vi "Read Test running.vi"(8 "error in (no error)":errorcluster, 11 "Fiber Auto Collimation state data in":refnum<class "Fiber Auto Collimation state data.lvclass">) -> (0 "error out":errorcluster, 2 "Test running":bool, 3 "Fiber Auto Collimation state data out":refnum<class "Fiber Auto Collimation state data.lvclass">, 4 "Disable control(s) when test is running":T1(ring))   [LabVIEW 2018, in "Fiber Auto Collimation state data.lvclass"]
doc: "A Boolean which should be set to True whenever a test is running, usually to disable a number of controls.\n\nThere is an output added to make it easier to disable controls when the test is running, which is a pretty common thing to do in the Model loop."
uses:
  Fiber Auto Collimation state data.lvclass
  Fiber Auto Collimation state data.lvclass/Fiber Auto Collimation state data.ctl
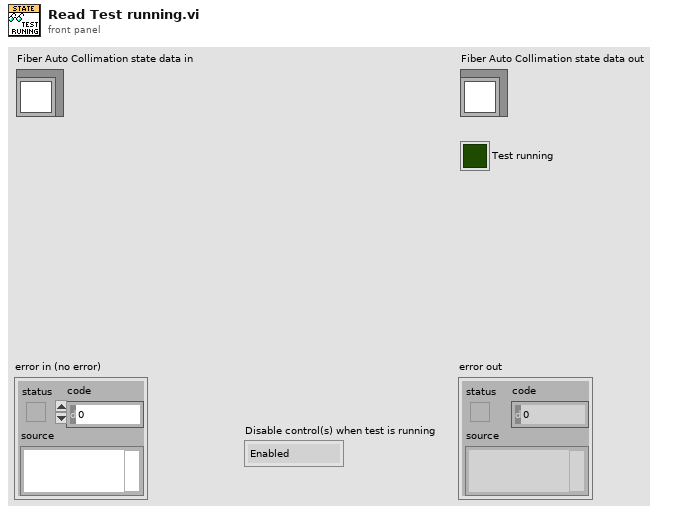
[diagram p1: front panel]
types:
  T1 = enum8{"Enabled", "Disabled", "Disabled and Grayed Out"}
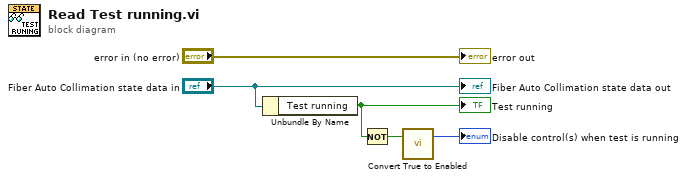
[diagram p0: block diagram]
diagram:
  n1 = Unbundle By Name("Fiber Auto Collimation state data in") -> ("Test running"=w3:bool)
  "Test running" <- w3
  n2 = Not(x=w3) -> (.not. x?=w2:bool)
  n3 = call <userlib>:"Convert True to Enabled.vi"("Enable?"=w2) -> ("Enabled"=→"Disable control(s) when test is running":T1)  [unwired: 2 in]
  "error out" <- "error in (no error)"
  "Fiber Auto Collimation state data out" <- "Fiber Auto Collimation state data in"
